vi "MC5e Save Squad XML.vi"(8 "error in":errorcluster, 10 "Cancelled?":bool, 11 "selected path":path) -> (0 "error out":errorcluster)   [LabVIEW 2020]
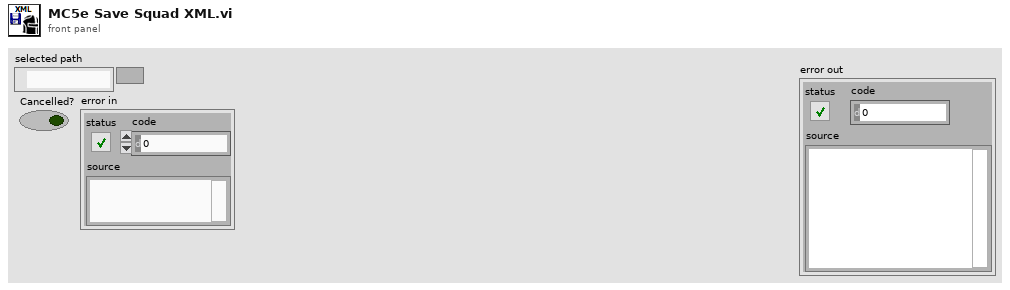
[diagram p1: front panel]
types:
  T1 = enum16{"open", "replace", "create", "open or create", "replace or create", "replace or create with confirmation"}
  T2 = typedef "MC5e Squad_Info.ctl" = cluster{"Squad Name":string, "# Soldiers":u16, "Battle Rating":u16, "Flying":bool, "Mounted":bool, "Speed":u16, "Range":u16, "Morale":i32, "Token Image":variant, "Max Endurance":u16, "Current Endurance":i32, "Size":T3, "Space Taken":u16, "Difficult Terrain":i32[], "CR":u16, "Special / Notes":string}
  T3 = typedef "MC5e Size_Categories.ctl" = enum16{"Tiny", "Small", "Medium", "Large", "Huge", "Gargantuan"}
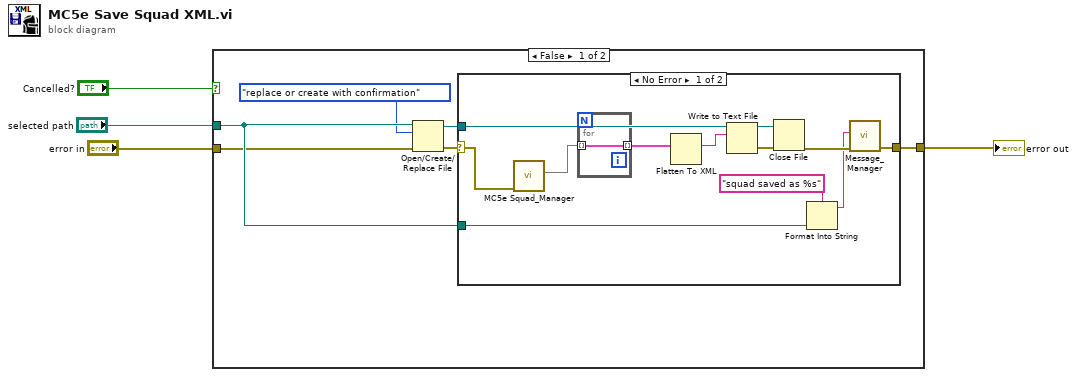
[diagram p0: block diagram]
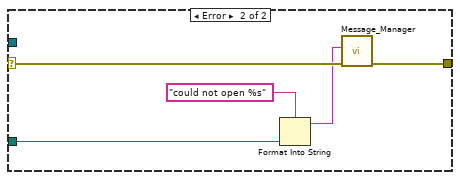
[diagram p2: hidden frame]
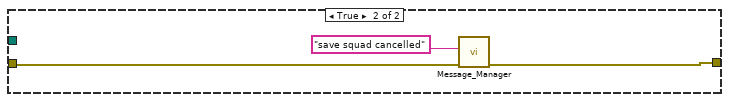
[diagram p3: hidden frame]
diagram:
  n1 = case shown="False" "Cancelled?" {
    tunnel: "selected path" -> [w10 _]
    tunnel: "error in" -> [w7 w31]
    tunnel: [w6 w29] -> w1
    frame False {
      n2 = Open/Create/Replace File(file path (use dialog)=w10, error in=w7, operation (0:open)=T1."replace or create with confirmation") -> (refnum out=w8:refnum<file>, error out=w9:errorcluster)  [unwired: 3 in, 1 out]
      n3 = case shown="No Error" w9 {
        selector: w9 -> [w12 w28]
        tunnel: w8 -> [w22 _]
        tunnel: [w18 w27] -> w6
        tunnel: w10 -> [w15 w25]
        frame No Error {
          n4 = call "MC5e Squad_Manager.vi"("error in"=w12) -> ("Set"=w13:set{T2})  [unwired: 7 in, 3 out]
          n5 = for {
            tunnel: w13 -> [w23] mode=indexing
            tunnel: [w23] -> w11 mode=indexing
          }
          n6 = Flatten To XML(6:w11) -> (2:w20:string)
          n7 = Write to Text File(file (use dialog)=w22, text=w20) -> (refnum out=w21:refnum<file>, error out=w19:errorcluster)  [unwired: 2 in, 1 out]
          n8 = Close File(refnum=w21, error in=w19) -> (error out=w17:errorcluster)  [unwired: 1 out]
          n9 = Format Into String(format string="squad saved as %s" ("New Entry"), w15) -> (resulting string=w14:string)  [unwired: 2 in, 1 out]
          n10 = call "Message_Manager.vi"("error in"=w17, "New Entry"=w14) -> ("error out"=w18:errorcluster)  [unwired: 5 in, 4 out]
        }
        frame Error {
          n11 = Format Into String(format string="could not open %s", w25) -> (resulting string=w24:string)  [unwired: 2 in, 1 out]
          n12 = call "Message_Manager.vi"("error in"=w28, "New Entry"=w24) -> ("error out"=w27:errorcluster)  [unwired: 5 in, 4 out]
        }
      }
    }
    frame True {
      n13 = call "Message_Manager.vi"("error in"=w31, "New Entry"="save squad cancelled") -> ("error out"=w29:errorcluster)  [unwired: 5 in, 4 out]
    }
  }
  "error out" <- w1
